vi "Application Globals.vi"() -> ()   [LabVIEW 2016]
uses:
  FSM States.ctl
  HostRTCommunication/Command and Parameters.ctl
  HostRTCommunication/Commands.ctl
panel:
  in  "Raw Data Queue":refnum<queue>
  in  "Command Writer":refnum<k21>
  in  "UISpectrumNotifier":refnum<notifier>
  in  "FSM Command Queue":refnum<queue>
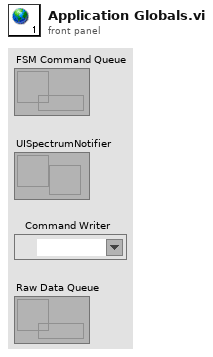
[diagram p1: front panel]
diagram:
